vi "Region-det-rel-queue.vi"(8 "error in (no error)":errorcluster, 11 "Queues":T1) -> (0 "error out":errorcluster)   [LabVIEW 2016]
uses:
  Sched_queues.ctl
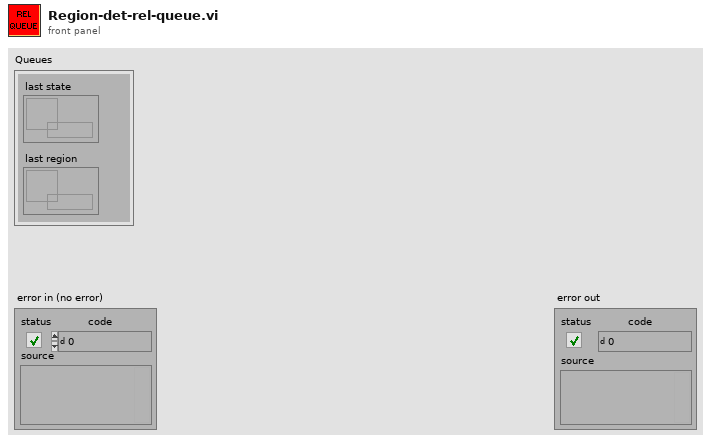
[diagram p1: front panel]
types:
  T1 = typedef "Sched_queues.ctl" = cluster{"last region":refnum<queue>, "last state":refnum<queue>}
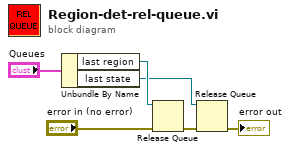
[diagram p0: block diagram]
diagram:
  n1 = Unbundle By Name("Queues") -> ("last region"=w5:refnum<queue>, "last state"=w4:refnum<queue>)
  n2 = Release Queue(queue=w5, error in (no error)="error in (no error)") -> (error out=w3:errorcluster)  [unwired: 1 in, 2 out]
  n3 = Release Queue(queue=w4, error in (no error)=w3) -> (error out=→"error out":errorcluster)  [unwired: 1 in, 2 out]
